vi "get Session Handle Queue.vi"(0 "OBJ - Session in":refnum<class "Sequence Automation Session.lvclass">, 11 "error in (no error)":errorcluster) -> (4 "OBJ - Session out":refnum<class "Sequence Automation Session.lvclass">, 6 "Session Queue Handle":refnum<queue>, 8 "Last Session?":bool, 15 "error out":errorcluster)   [LabVIEW 2018, in "Sequence Automation Session.lvlib" / "Sequence Automation Session.lvclass"]
doc: "Extracts named notifier; typically to release or destroy reference"
uses:
  Sequence Automation Session.lvclass
  Sequence Automation Session.lvclass/Sequence Automation Session.ctl
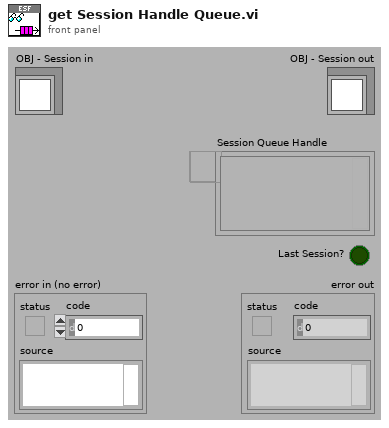
[diagram p1: front panel]
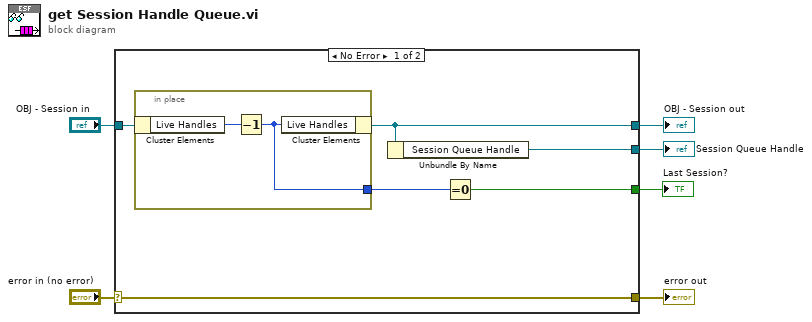
[diagram p0: block diagram]
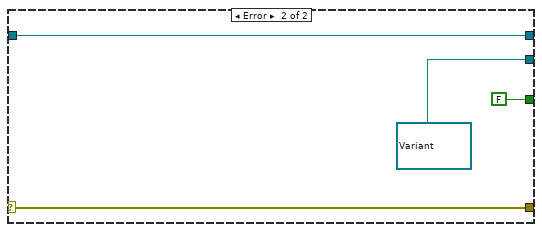
[diagram p2: hidden frame]
diagram:
  n1 = case shown="No Error" "error in (no error)" {
    selector: "error in (no error)" -> [w12 w17]
    tunnel: [w12 w17] -> w5
    tunnel: [w8 w18] -> w3
    tunnel: "OBJ - Session in" -> [w11 w18]
    tunnel: [w7 refnum<queue> refnum ("Session Queue Handle")] -> w2
    tunnel: [w9 FALSE] -> w1
    frame No Error {
      n2 = in-place {
        in-place-border: [w13] -> w10
        n3 = in-place-cluster #1(w11) -> ("Live Handles"=w14:u32)
        n4 = Decrement(x=w14) -> (x-1=w13:u32)
        n5 = in-place-cluster #1("Live Handles"=w13) -> (w8:refnum<class "Sequence Automation Session.lvclass">)
      }
      n6 = Unbundle By Name(w8) -> ("Session Queue Handle"=w7:refnum<queue>)
      n7 = Equal To 0?(x=w10) -> (x = 0?=w9:bool)
    }
    frame Error {
    }
  }
  "error out" <- w5
  "OBJ - Session out" <- w3
  "Session Queue Handle" <- w2
  "Last Session?" <- w1
